vi "Motic Get Frequency Count.vi"(8 "error in (no error)":errorcluster, 11 "camera":i32) -> (0 "error out":errorcluster, 2 "frequency count":i32, 3 "camera out":i32)   [LabVIEW 2012, in "MoticApi.lvlib"]
doc: "MOTICAPI int Motic_GetFrequencyCount(MUCam_Handle camera);"
uses:
  MoticApi.lvlib
  MoticApi.dll
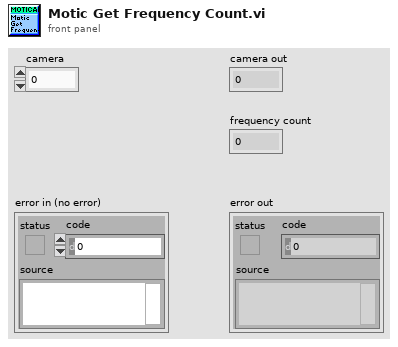
[diagram p1: front panel]
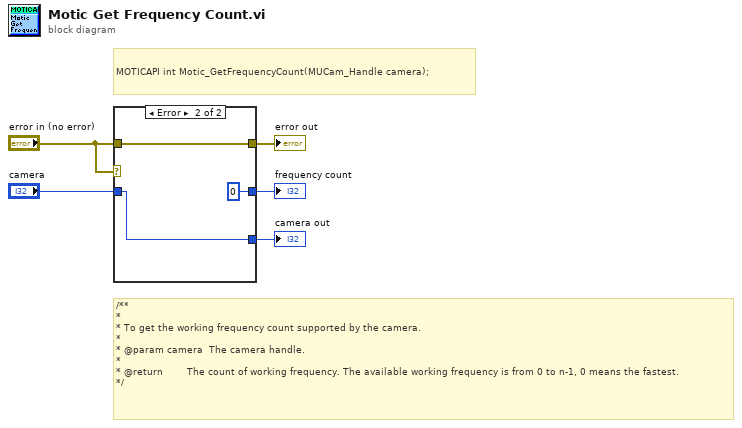
[diagram p0: block diagram]
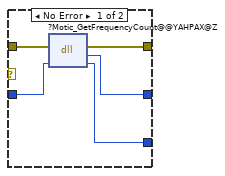
[diagram p2: hidden frame]
diagram:
  # "/**\n*\n* To get the working frequency count supported by the camera.\n*\n* @param camera  The camera handle.\n*\n* @return        The count of working frequency. The available working frequency is from 0 to n-1, 0 means the fastest.\n*/"
  # "MOTICAPI int Motic_GetFrequencyCount(MUCam_Handle camera);"
  n1 = case shown="Error" "error in (no error)" {
    tunnel: [w10 0] -> w5
    tunnel: "camera" -> [w9 w12]
    tunnel: [w8 w12] -> w3
    tunnel: "error in (no error)" -> [w7 w13]
    tunnel: [w6 w13] -> w2
    frame No Error {
      n2 = dll-call lib="C:/Users/TTS-Digital/Desktop/MoticApi/MoticApi_git/MoticApi/MoticApi.*" fn="?Motic_GetFrequencyCount@@YAHPAX@Z"(error in=w7, "camera"=w9) -> (error out=w6:errorcluster, w10:i32, "camera"=w8:i32)  [unwired: 2 in, 1 out]
    }
    frame Error {
    }
  }
  "frequency count" <- w5
  "camera out" <- w3
  "error out" <- w2
